vi "Teleop Elevator Control.vi"(8 "Button Cluster":T2, 9 "Driver Joystick":T3, 10 "Call Context":T1, 11 "Manipulator Joystick":T3) -> ()   [LabVIEW 2014]
uses:
  <vilib>/Rock Robotics/WPI/Joystick/WPI_JoystickDevRef.ctl
  <vilib>/Rock Robotics/WPI/Joystick/WPI_JoystickDeviceEnum.ctl
  Real-Life Controls/Button Cluster.ctl
  <vilib>/Rock Robotics/WPI/DriverStation/WPI_DriverStationDerivedRobotMode.ctl
  Elevator Control Command.ctl
  Elevator Command.ctl
  Common Code/Elevator Mode.ctl
  Common Code/Elevator Idle Mode.ctl
  Common Code/Elevator State.ctl
  Common Code/Change Detect Int.vi
  Common Code/Change Detect Boolean.vi
  Robot Global Data.vi
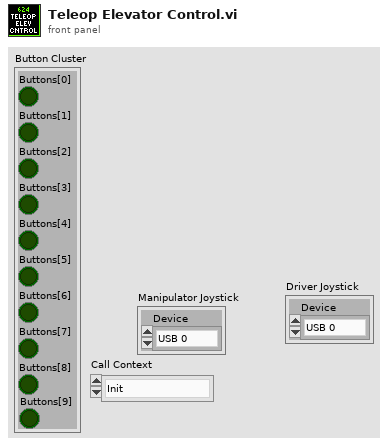
[diagram p1: front panel]
types:
  T1 = typedef "WPI_DriverStationDerivedRobotMode.ctl" = enum16{"Init", "Execute", "Stop"}
  T2 = typedef "Button Cluster.ctl" = cluster{"Buttons[0]":bool, "Buttons[1]":bool, "Buttons[2]":bool, "Buttons[3]":bool, "Buttons[4]":bool, "Buttons[5]":bool, "Buttons[6]":bool, "Buttons[7]":bool, "Buttons[8]":bool, "Buttons[9]":bool}
  T3 = typedef "WPI_JoystickDevRef.ctl" = cluster{"Device":T4}
  T4 = typedef "WPI_JoystickDeviceEnum.ctl" = enum16{"USB 0", "USB 1", "USB 2", "USB 3", "USB 4", "USB 5"}
  T5 = enum16{"0", "1", "2", "3", "4", "5", "6", "7", "8", "9", "A", "B", "C", "D", "E", "F", "G", "H", "I", "J", "K", "L", "M", "N", "O", "P", "Q", "R", "S", "T", "U", "V", "W", "X", "Y", "Z", "F1", "F2", "F3", "F4", "F5", "F6", "F7", "F8", "F9", "F10", "F11", "F12", "F13", "F14", "F15", "ADD", "BACK", "BACKSLASH", "CAPITAL", "COMMA", "DECIMAL", "DELETE", "DIVIDE", "DOWN", "END", "EQUALS", "ESCAPE", "GRAVE (`)", "HOME", "INSERT", "LBRACKET", "LCONTROL", "LEFT", "L ALT", "LSHIFT", "LWIN", "MINUS", "MULTIPLY", "NEXT", "NUMLOCK", "NUMPAD_0", "NUMPAD_1", "NUMPAD_2", "NUMPAD_3", "NUMPAD_4", "NUMPAD_5", "NUMPAD_6", "NUMPAD_7", "NUMPAD_8", "NUMPAD_9", "PAUSE", "PERIOD", "PRIOR (PG UP)", "RBRACKET", "RCONTROL", "RETURN", "RIGHT", "R ALT", "RSHIFT", "RWIN", "SCROLL", "SEMICOLON", "SLASH", "SPACE", "SUBTRACT", "TAB", "UP", "ENTER (num pad)", "' (quote)"}
  T6 = typedef "Elevator Control Command.ctl" = cluster{"Command":T7, "Manual Motor Out":dbl, "Manual Eject Piston":bool, "Mode":T8, "Override Limits":bool, "Manual Stabilizer":bool, "Manual Finger":bool, "Store Trashcan?":bool, "Hold Low?":bool, "Idle Mode":T9, "HP Load":bool, "Unstick":bool, "Raw Height Set":dbl, "Force Store":bool}
  T7 = typedef "Elevator Command.ctl" = enum16{"Idle", "Load 1", "Load 2", "Load 3", "Drop Stack", "Eject Stack", "Untip Trashcan", "Load Trashcan", "HP Load", "HP Score"}
  T8 = typedef "Elevator Mode.ctl" = enum16{"Manual", "Safe", "Auto"}
  T9 = typedef "Elevator Idle Mode.ctl" = enum16{"Load 1", "Load 2", "Load 3", "Load Can", "Untip Can", "Step Load", "Drop Stack", "Raw Height"}
  T10 = typedef "Elevator Status.ctl" = cluster{"Height":dbl, "Enc Value":dbl, "Limit Override":bool, "Mode":T8, "High IR":bool, "Motor Out":dbl, "Ping Detect":bool, "Auto Elevator Indicators":T11, "Master Current":dbl, "Slave Current":dbl, "High Current":bool, "Current Tripped":bool, "Top Limit":bool, "Bottom Limit":bool, "Eject Piston":bool, "Stabilizer":bool, "Finger":bool, "Finger Height":dbl, "Finger Raw":dbl, "Finger at Bottom":bool}
  T11 = typedef "Auto Elevator Indicators.ctl" = cluster{"Target Out":dbl, "Storing Trashcan?":bool, "State":T12, "In Range":bool, "Store Can Command":bool, "HP Load":bool}
  T12 = typedef "Elevator State.ctl" = enum16{"Idle", "Goto Load Position", "Wait for Load", "Load Drop", "Load Lift", "Drop Stack", "Goto Eject Position", "Eject ", "Raise Trashcan", "Open Stabilizer", "Untip Drop", "Untip Wait", "Untip Lift", "Abort Load", "HP Load Wait", "HP Load Drop", "HP Load Lift", "HP Load Abort", "Close Stabilizer", "HP Load Unfinish", "HP Load Score", "HP Load Finish", "HP Goto Finish Down", "HP Goto Finish Up", "Full"}
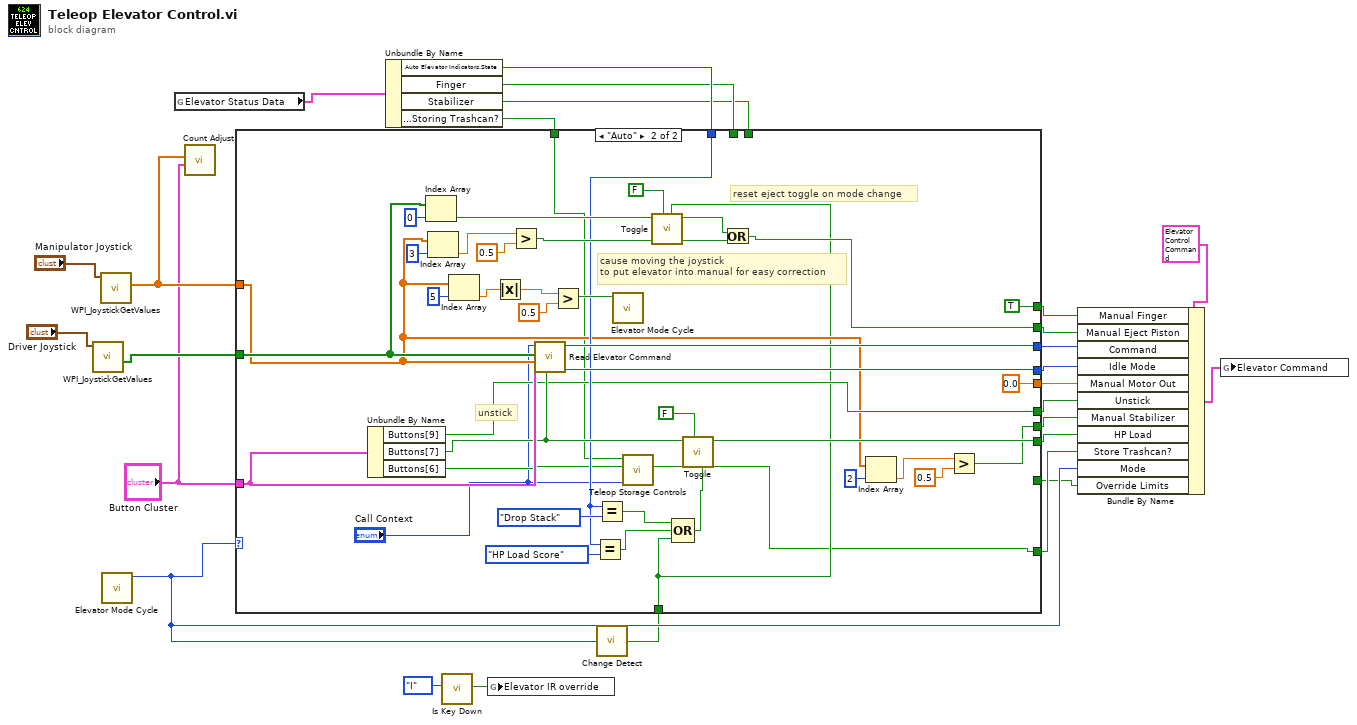
[diagram p0: block diagram]
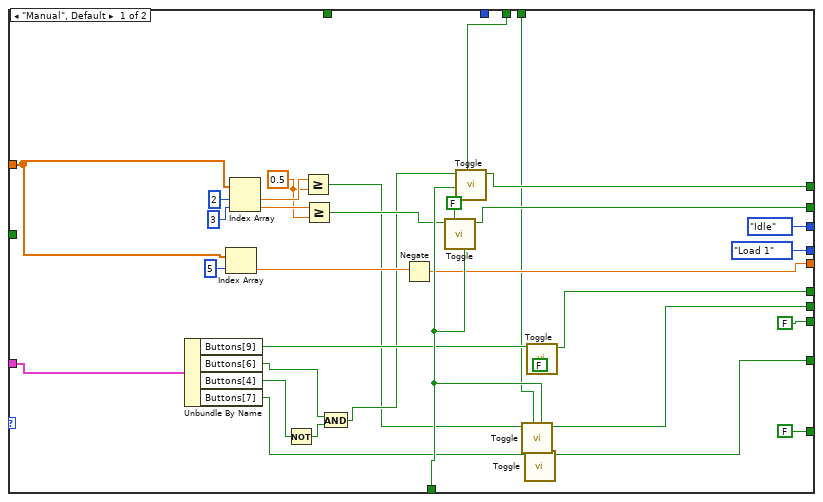
[diagram p2: hidden frame]
diagram:
  n1 = call <vilib>:"WPI_JoystickGetValues.vi"("JoystickDevRef"="Driver Joystick") -> ("Buttons"=w14:bool[])  [unwired: 6 in, 4 out]
  n2 = call <vilib>:"WPI_JoystickGetValues.vi"("JoystickDevRef"="Manipulator Joystick") -> ("Axes"=w10:dbl[])  [unwired: 6 in, 4 out]
  n3 = call "Elevator Mode Cycle.vi"() -> ("Mode"=w4:T8)  [unwired: 11 in]
  n4 = global read "Robot Global Data.vi" "Elevator Status Data"() -> (w5:T10)
  n5 = call "Count Adjust.vi"("Button Cluster"="Button Cluster", "Axes"=w10) -> ()  [unwired: 10 in]
  n6 = Unbundle By Name(w5) -> ("Auto Elevator Indicators.State"=w8:T12, "Finger"=w7:bool, "Stabilizer"=w6:bool, "Auto Elevator Indicators.Storing Trashcan?"=w3:bool)
  n7 = call "Is Key Down.vi"("Key"=T5."I") -> ("Key Down?"=w24:bool)  [unwired: 10 in]
  n8 = global write "Robot Global Data.vi" "Elevator IR override"(w24) -> ()
  n9 = call-poly "Change Detect.vi"("In"=w4) -> ("Changed?"=w2:bool)
  n10 = case shown="\"Auto\"" w4 {
    tunnel: "Button Cluster" -> [w49 w95]
    tunnel: w14 -> [_ w93]
    tunnel: w10 -> [w53 w67]
    tunnel: [w58 w77] -> w20
    tunnel: [Elevator_Command."Idle" ("Command") w96] -> w13
    tunnel: [Elevator_Idle_Mode."Load 1" ("Idle Mode") w97] -> w12
    tunnel: [FALSE ("Toggled") w60] -> w15
    tunnel: [w56 TRUE ("Toggled")] -> w22
    tunnel: w2 -> [w57 w64]
    tunnel: w8 -> [_ w74]
    tunnel: [w50 0.0] -> w19
    tunnel: [w46 w73] -> w17
    tunnel: [w47 w65] -> w18
    tunnel: w7 -> [w31 _]
    tunnel: [FALSE ("Toggled") w94] -> w16
    tunnel: w6 -> [w32 _]
    tunnel: w3 -> [_ w63]
    tunnel: [w27 _] -> w1
    frame "Manual", Default {
      w41 = 0.5 ("y")
      n11 = Unbundle By Name(w49) -> ("Buttons[9]"=w48:bool, "Buttons[6]"=w34:bool, "Buttons[4]"=w35:bool, "Buttons[7]"=w28:bool)
      n12 = Index Array(array=w53, index=5) -> (element=w52:dbl)
      n13 = Index Array(array=w53, index #1=2 ("index"), index #2=3 ("index")) -> (element #1=w55:dbl, element #2=w54:dbl)
      n14 = Not(x=w35) -> (.not. x?=w33:bool)
      n15 = Greater Or Equal?(x=w55, y=w41) -> (x >= y?=w29:bool)
      n16 = Greater Or Equal?(x=w54, y=w41) -> (x >= y?=w42:bool)
      n17 = And(x=w34, y=w33) -> (x .and. y?=w30:bool)
      n18 = Negate(x=w52) -> (-x=w50:dbl)
      n19 = call "Toggle.vi"("Reinit?"=w57, "Initial Value"=FALSE, "In"=w42) -> ("Toggled"=w58:bool)  [unwired: 8 in]
      n20 = call "Toggle.vi"("Reinit?"=w57, "Initial Value"=w31, "In"=w30) -> ("Toggled"=w56:bool)  [unwired: 8 in]
      n21 = call "Toggle.vi"("Reinit?"=w57, "Initial Value"=w32, "In"=w29) -> ("Toggled"=w47:bool)  [unwired: 8 in]
      n22 = call "Toggle.vi"("In"=w28) -> ("Toggled"=w27:bool)  [unwired: 10 in]
      n23 = call "Toggle.vi"("Initial Value"=FALSE, "In"=w48) -> ("Toggled"=w46:bool)  [unwired: 9 in]
    }
    frame "Auto" {
      # "unstick"
      # "reset eject toggle on mode change"
      # "cause moving the joystick \nto put elevator into manual for easy correction"
      n24 = Unbundle By Name(w95) -> ("Buttons[9]"=w73:bool, "Buttons[7]"=w76:bool, "Buttons[6]"=w62:bool)
      n25 = Index Array(array=w93, index=0) -> (element=w79:bool)
      n26 = Index Array(array=w67, index=3) -> (element=w80:dbl)
      n27 = Index Array(array=w67, index=5) -> (element=w82:dbl)
      n28 = Absolute Value(x=w82) -> (abs(x)=w89:dbl)
      n29 = Greater?(x=w80, y=0.5) -> (0:w84:bool)
      n30 = call "Read Elevator Command.vi"("Reset Idle State"=w76, "Button Cluster"=w95, "Axes"=w67, "Driver Buttons"=w93, "Call Context"="Call Context") -> ("Idle Mode"=w97:T9, "Command"=w96:T7)  [unwired: 5 in]
      n31 = Greater?(x=w89, y=0.5) -> (0:w87:bool)
      n32 = Equal?(x=w74, y=Elevator_State."HP Load Score" ("Auto Elevator Indicators.State")) -> (x = y?=w71:bool)
      n33 = Equal?(x=w74, y=Elevator_State."Drop Stack") -> (x = y?=w72:bool)
      n34 = call "Elevator Mode Cycle.vi"("Set to Manual"=w87) -> ()  [unwired: 10 in, 1 out]
      n35 = call "Teleop Storage Controls.vi"("Call Context"="Call Context", "Store Button"=w62, "Storing Can?"=w63) -> ("Store Can?"=w60:bool)  [unwired: 8 in]
      n36 = call "Toggle.vi"("Reinit?"=w64, "Initial Value"=FALSE, "In"=w79) -> ("Toggled"=w78:bool)  [unwired: 8 in]
      n37 = Compound Arithmetic op=OR(w72, w71, w64) -> (w70:bool)
      n38 = call "Toggle.vi"("Reinit?"=w70, "Initial Value"=FALSE, "In"=w76) -> ("Toggled"=w94:bool)  [unwired: 8 in]
      n39 = Or(x=w78, y=w84) -> (x .or. y?=w77:bool)
      n40 = Index Array(array=w67, index=2) -> (element=w66:dbl)
      n41 = Greater?(x=w66, y=0.5) -> (0:w65:bool)
    }
  }
  n42 = Bundle By Name(cluster=T6 {"Command"=enum."Idle", "Manual Motor Out"=0.0, "Manual Eject Piston"=FALSE, "Mode"=enum."Manual", "Override Limits"=FALSE, "Manual Stabilizer"=FALSE, "Manual Finger"=FALSE, "Store Trashcan?"=FALSE, "Hold Low?"=FALSE, "Idle Mode"=enum."Load Can", "HP Load"=FALSE, "Unstick"=FALSE, "Raw Height Set"=0.0, "Force Store"=FALSE} ("Elevator Command"), "Manual Finger"=w22, "Manual Eject Piston"=w20, "Command"=w13, "Idle Mode"=w12, "Manual Motor Out"=w19, "Unstick"=w17, "Manual Stabilizer"=w18, "HP Load"=w16, "Store Trashcan?"=w15, "Mode"=w4, "Override Limits"=w1) -> (w21:T6)
  n43 = global write "Robot Global Data.vi" "Elevator Command"(w21) -> ()
